vi "Accumulator.vi"(10 "Reset?":bool, 11 "Value":dbl) -> (3 "Sum":dbl)   [LabVIEW 2019]
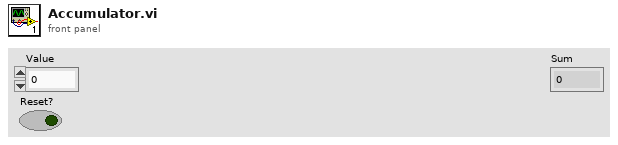
[diagram p1: front panel]
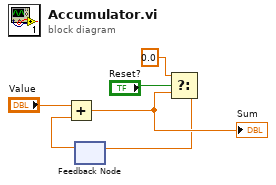
[diagram p0: block diagram]
diagram:
  n1 = feedback #1() -> (w6:dbl)  [unwired: 1 in]
  n2 = Add(x="Value", y=w6) -> (x+y=w2:dbl)
  "Sum" <- w2
  n3 = Select(t=0.0, s="Reset?", f=w2) -> (s? t:f=w1:dbl)
  n4 = feedback-in #1(w1) -> ()
